vi "util.load.u64.from.array.vi"(11 "Data.in":u8[](array[numeric])) -> (2 "Numeric":u64, 3 "Data.out":u8[](array[numeric]))   [LabVIEW 2021]
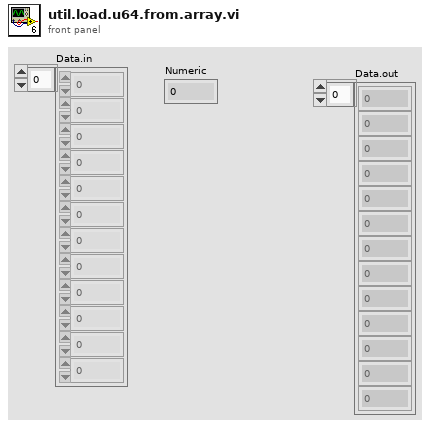
[diagram p1: front panel]
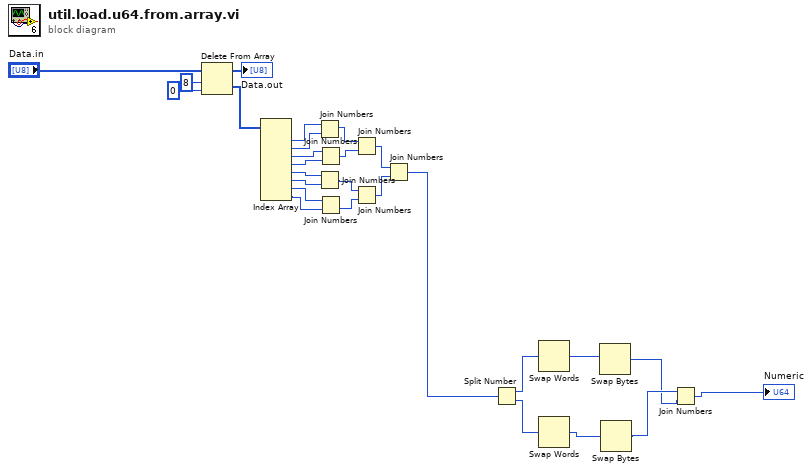
[diagram p0: block diagram]
diagram:
  n1 = Delete From Array(array="Data.in", length=8, index=0) -> (deleted portion=w3:u8[], array with subset deleted=→"Data.out":u8[])
  n2 = Index Array(array=w3) -> (element #1=w14:u8, element #2=w15:u8, element #3=w16:u8, element #4=w17:u8, element #5=w18:u8, element #6=w19:u8, element #7=w20:u8, element #8=w21:u8)  [unwired: 8 in]
  n3 = Join Numbers(hi=w14, lo=w15) -> ((hi.lo)=w22:u16)
  n4 = Join Numbers(hi=w18, lo=w19) -> ((hi.lo)=w24:u16)
  n5 = Join Numbers(hi=w16, lo=w17) -> ((hi.lo)=w23:u16)
  n6 = Join Numbers(hi=w20, lo=w21) -> ((hi.lo)=w25:u16)
  n7 = Join Numbers(hi=w22, lo=w23) -> ((hi.lo)=w27:u32)
  n8 = Join Numbers(hi=w24, lo=w25) -> ((hi.lo)=w26:u32)
  n9 = Join Numbers(hi=w27, lo=w26) -> ((hi.lo)=w7:u64)
  n10 = Split Number(x=w7) -> (hi(x)=w13:u32, lo(x)=w12:u32)
  n11 = Swap Words(1:w13) -> (0:w11:u32)
  n12 = Swap Words(1:w12) -> (0:w10:u32)
  n13 = Swap Bytes(anything=w11) -> (byte swapped=w8:u32)
  n14 = Swap Bytes(anything=w10) -> (byte swapped=w9:u32)
  n15 = Join Numbers(hi=w9, lo=w8) -> ((hi.lo)=→"Numeric":u64)
